vi "create restart acquisition loop command.vi"() -> (3 "command message":variant)   [LabVIEW 2018]
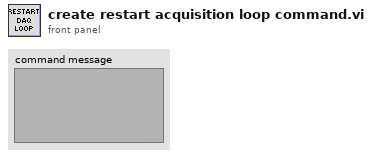
[diagram p1: front panel]
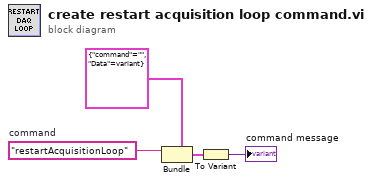
[diagram p0: block diagram]
diagram:
  w3 = "restartAcquisitionLoop"  # command
  n1 = Bundle(cluster=cluster{"command":string, "Data":variant} {"command"="", "Data"=variant}, "command"=w3) -> (w2:cluster{"command":string, "Data":variant})  [unwired: 1 in]
  n2 = To Variant(anything=w2) -> (Variant=→"command message":variant)
